vi "PFI-28000-Chan-28144-V_Get Shunt Connection.vi"(8 "error in (no error)":errorcluster, 11 "PFI-28000-Chan-28144-V in":refnum<class "PFI-28000-Chan-28144-V.lvclass">) -> (0 "error out":errorcluster, 2 "Shunt Connection":T1, 3 "PFI-28000-Chan-28144-V out":refnum<class "PFI-28000-Chan-28144-V.lvclass">)   [LabVIEW 2017, in "PFI-28000-Chan-28144-V.lvclass"]
uses:
  PFI-28000-Chan-28144-V.lvclass
  C:/wc/07143 Precision Filters 28000 Support/Driver/source/Channel/PFI-28000-Channel.lvclass
  PFI-28000-Chan-28144-V-Shunt Connection.ctl
  Utilities/PFI-28000-Utils.lvlib
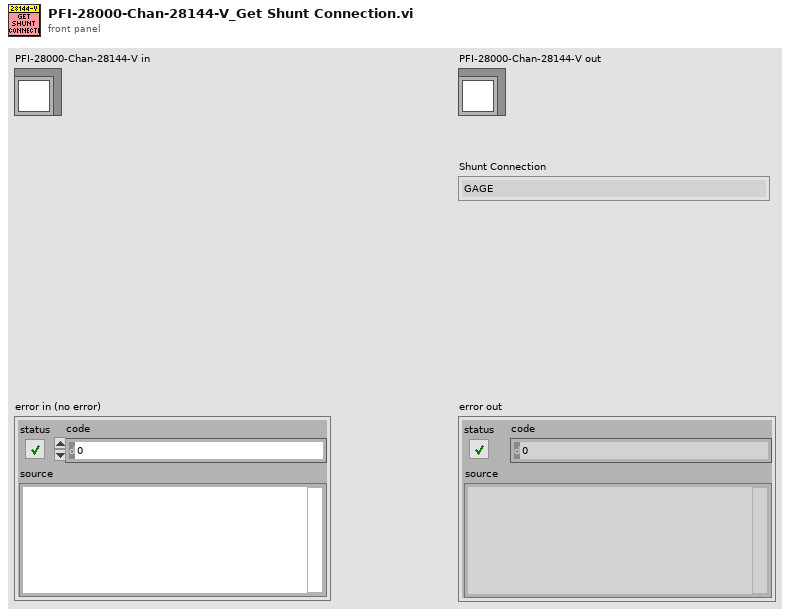
[diagram p1: front panel]
types:
  T1 = typedef "PFI-28000-Chan-28144-V.lvclass/PFI-28000-Chan-28144-V-Shunt Connection.ctl" = enum8{"GAGE", "INST"}
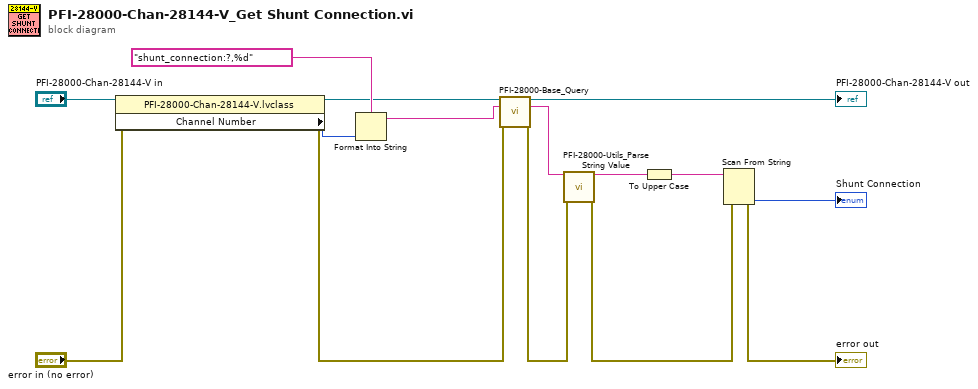
[diagram p0: block diagram]
diagram:
  n1 = property class="PFI-28000-Chan-28144-V.lvclass"(reference="PFI-28000-Chan-28144-V in", error in="error in (no error)") -> (reference out=w9:refnum<class "PFI-28000-Chan-28144-V.lvclass">, error out=w5:errorcluster, "Channel Number"=w13:i32)
  n2 = Format Into String(format string="shunt_connection:?,%d" ("empty string"), w13) -> (resulting string=w7:string)  [unwired: 2 in, 1 out]
  n3 = call-dynamic "PFI-28000-Base_Query.vi"("PFI-28000-Base in"=w9, "Command"=w7, "error in (no error)"=w5) -> ("PFI-28000-Base out"=→"PFI-28000-Chan-28144-V out":refnum<class "PFI-28000-Chan-28144-V.lvclass">, "Response"=w3:string, "error out"=w4:errorcluster)  [unwired: 9 in, 1 out]
  n4 = call "PFI-28000-Utils_Parse String Value.vi"("String"=w3, "error in (no error)"=w4) -> ("String Value"=w2:string, "error out"=w6:errorcluster)  [unwired: 11 in, 1 out]
  n5 = To Upper Case(1:w2) -> (0:w1:string)
  n6 = Scan From String(input string=w1, error in=w6) -> (error out=→"error out":errorcluster, output 1=→"Shunt Connection":T1)  [unwired: 3 in, 2 out]
